vi "Wirtualny Przełącznik.vi"() -> ()   [LabVIEW 2020]
panel:
  in  "?":bool
  in  "Third":bool
  in  "Second":bool
  in  "Primo":bool
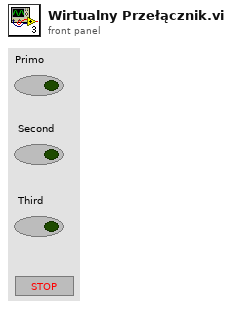
[diagram p1: front panel]
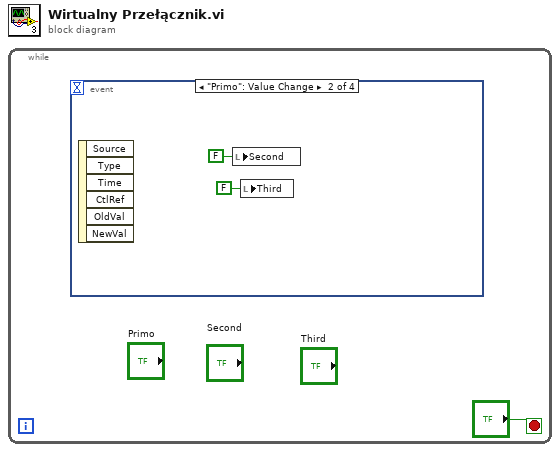
[diagram p0: block diagram]
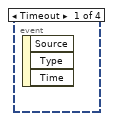
[diagram p2: hidden frame]
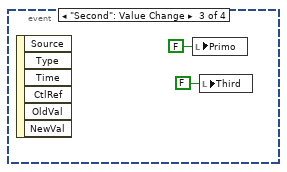
[diagram p3: hidden frame]
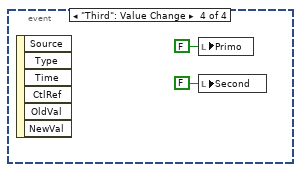
[diagram p4: hidden frame]
diagram:
  n1 = while {
    stop <- "?" stop-if-true
    n2 = event shown="[1] \"Primo\": Value Change" {
      selector: _ -> [_ _ _ _]
      dyn-events: _ -> [_ _ _ _]
      timeout: _ -> [_ _ _ _]
      event Timeout {
        n3 = event-data() -> ()  [unwired: 1 in, 3 out]
      }
      event "Primo": Value Change {
        n4 = event-data() -> ()  [unwired: 1 in, 6 out]
        n5 = local write "Second"(FALSE ("Second")) -> ()
        n6 = local write "Third"(FALSE ("Third")) -> ()
      }
      event "Second": Value Change {
        n7 = event-data() -> ()  [unwired: 1 in, 6 out]
        n8 = local write "Primo"(FALSE ("Primo")) -> ()
        n9 = local write "Third"(FALSE ("Third")) -> ()
      }
      event "Third": Value Change {
        n10 = event-data() -> ()  [unwired: 1 in, 6 out]
        n11 = local write "Primo"(FALSE ("Primo")) -> ()
        n12 = local write "Second"(FALSE ("Second")) -> ()
      }
    }
  }
